vi "IP_ToHexString.vi"(11 "string":string) -> (3 "hex string":string)   [LabVIEW 2014, in "hse-network.lvlib"]
doc: "(v0.2.1b; 2017-08-14 16:44)\n\n\n\n____\nHAMPEL SOFTWARE ENGINEERING v0.7.0 (2018-07-16 18:12)"
uses:
  hse-network.lvlib
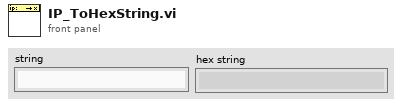
[diagram p1: front panel]
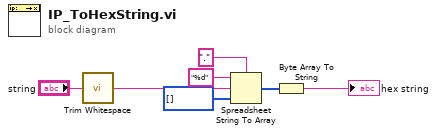
[diagram p0: block diagram]
diagram:
  n1 = call <vilib>:"Trim Whitespace.vi"("string"="string") -> ("trimmed string"=w3:string)  [unwired: 1 in]
  n2 = Spreadsheet String To Array(delimiter (Tab)=".", format string="%d", spreadsheet string=w3, array type (2D Dbl)=u8[] []) -> (array=w7:u8[])
  n3 = Byte Array To String(unsigned byte array=w7) -> (string=→"hex string":string)
